vi "Create Configuration List.vi"(0 "VISA resource name":refnum<visa-resource-name>, 5 "List Name":string="MyMeasList", 11 "error in (no error)":errorcluster) -> (4 "VISA resource name out":refnum<visa-resource-name>, 15 "error Out (no error)":errorcluster)   [LabVIEW 2021, in "Keithley DMM7510.lvlib"]
doc: "This VI creates an empty measure configuration list."
uses:
  Keithley DMM7510.lvlib
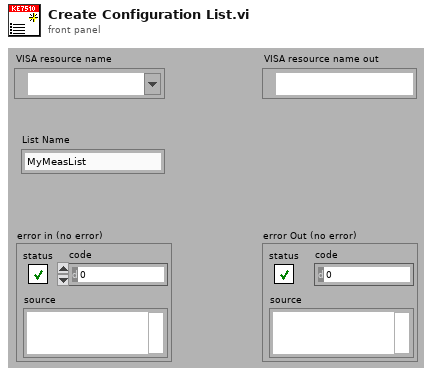
[diagram p1: front panel]
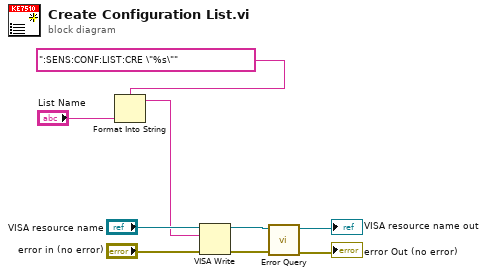
[diagram p0: block diagram]
diagram:
  n1 = Format Into String(format string=":SENS:CONF:LIST:CRE \"%s\"", "List Name") -> (resulting string=w6:string)  [unwired: 2 in, 1 out]
  n2 = VISA Write(VISA resource name="VISA resource name", write buffer=w6, error in (no error)="error in (no error)") -> (VISA resource name out=w5:refnum<visa-resource-name>, error out=w4:errorcluster)  [unwired: 1 out]
  n3 = call "Error Query.vi"("error in (no error)"=w4, "VISA resource name"=w5) -> ("error out"=→"error Out (no error)":errorcluster, "VISA resource name out"=→"VISA resource name out":refnum<visa-resource-name>)  [unwired: 6 in, 2 out]
